vi "Manager.vi"(7 "Action":T1, 8 "Error In":errorcluster, 11 "Set Value":variant) -> (0 "Error Out":errorcluster)   [LabVIEW 2017, in "Logger.lvlib" / "File.lvlib"]
uses:
  File.lvlib
  Action.ctl
  Public/Controls/Statement.ctl
  Public/Controls/Tag.ctl
  Create ISO 8601 File Name.vi
  Write Header.vi
  Create Calendar Folder Tree.vi
  Get Oldest File.vi
  <vilib>/Utility/libraryn.llb/Check if File or Folder Exists.vi
  Create Bulk CSV String.vi
  Logger.lvlib
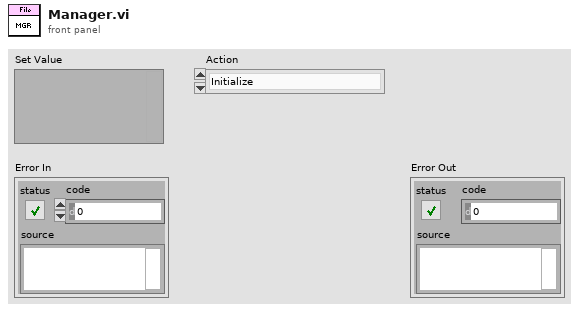
[diagram p1: front panel]
types:
  T1 = typedef "Logger.lvlib/File.lvlib/Action.ctl" = enum16{"Initialize", "Set Maximum File Size", "Set Maximum File Count", "Set Root Folder", "Set Enable Calendar Folder Tree", "Set File Extension", "Start", "Write", "Stop", "Shutdown"}
  T2 = typedef "Logger.lvlib/Statement.ctl" = cluster{"Time Stamp":timestamp, "Tag":T3, "Source":string, "Message":string}
  T3 = typedef "Logger.lvlib/Tag.ctl" = enum16{"Fatal", "Error", "Warn", "Info", "Debug", "Trace"}
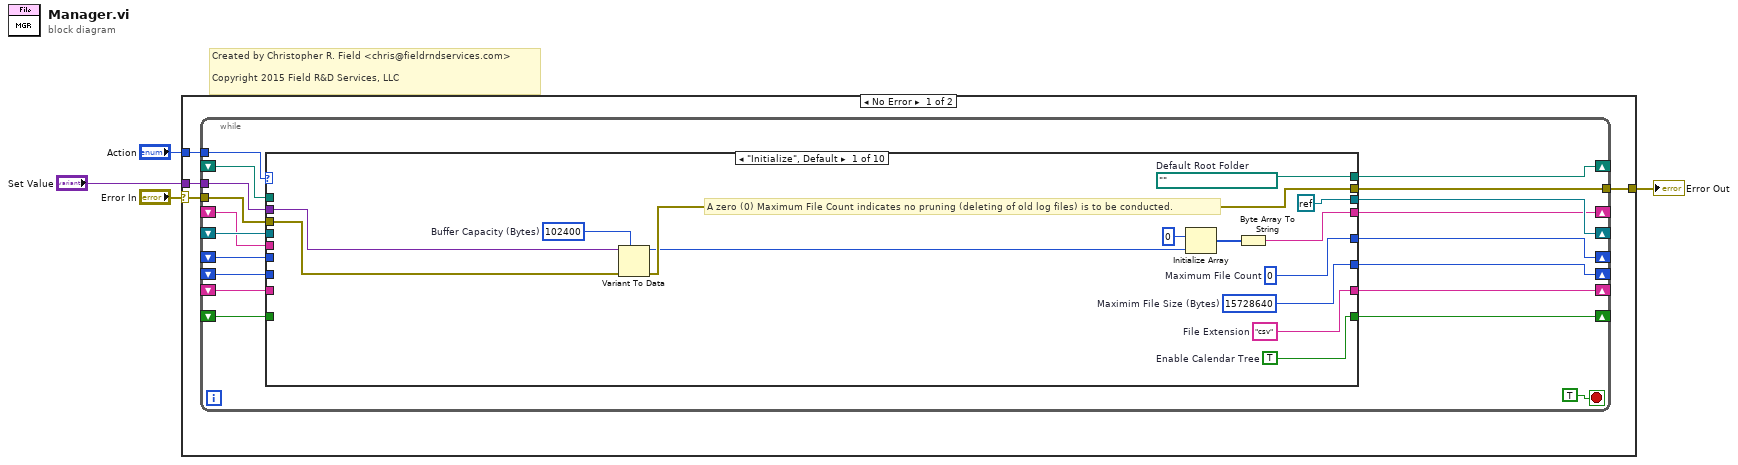
[diagram p0: block diagram]
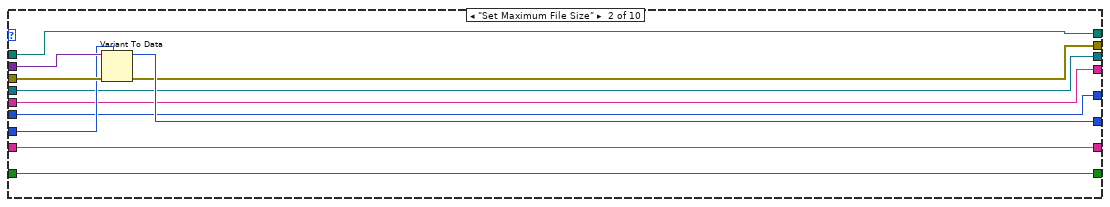
[diagram p2: hidden frame]
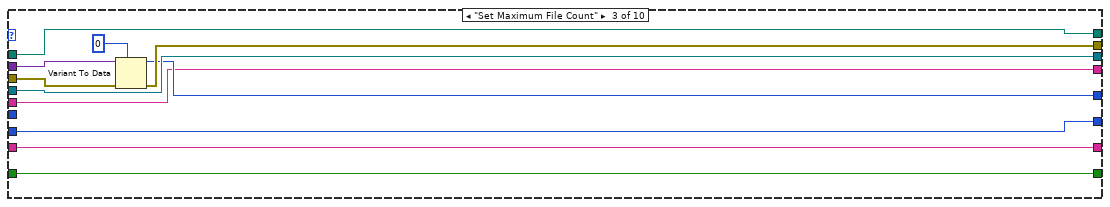
[diagram p3: hidden frame]
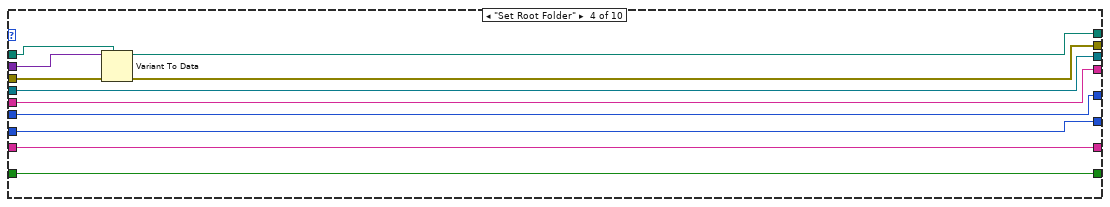
[diagram p4: hidden frame]
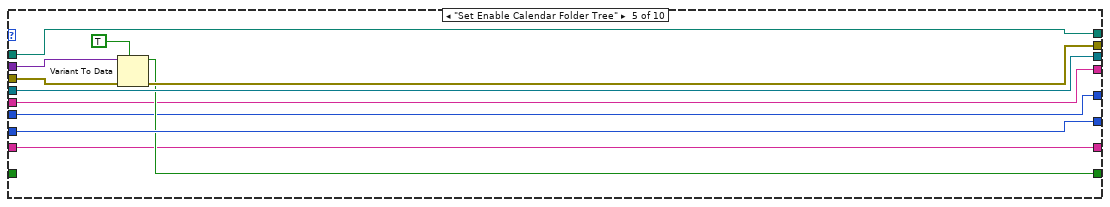
[diagram p5: hidden frame]
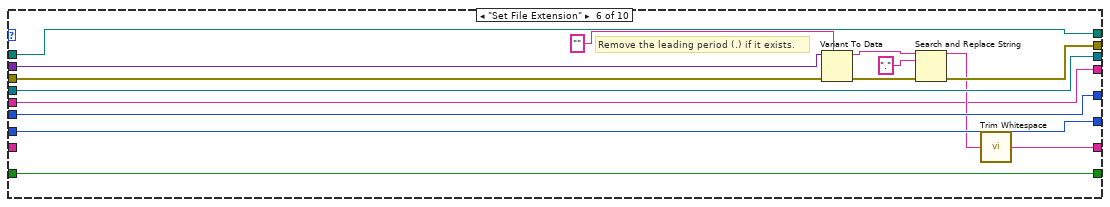
[diagram p6: hidden frame]
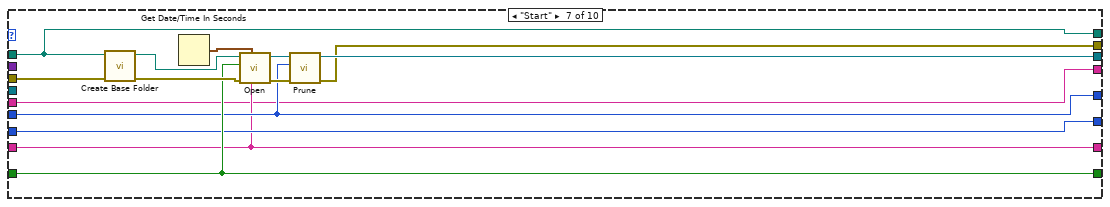
[diagram p7: hidden frame]
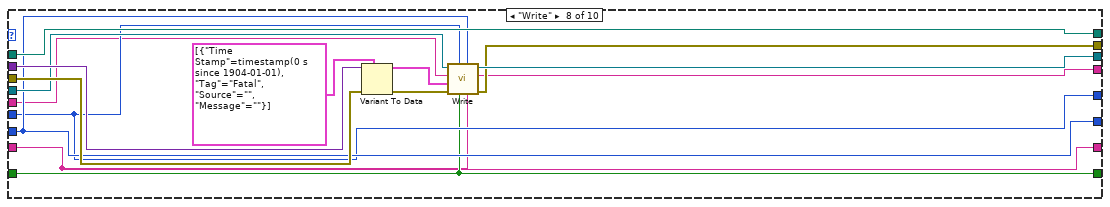
[diagram p8: hidden frame]
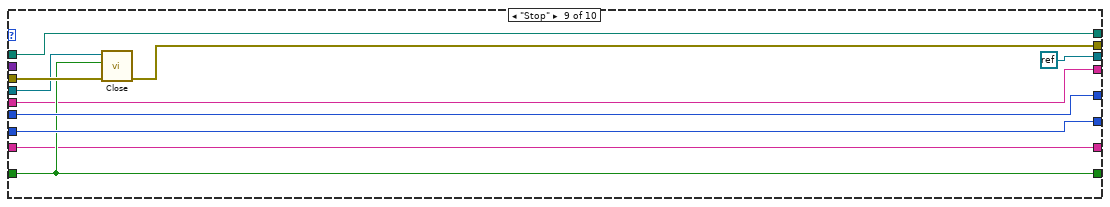
[diagram p9: hidden frame]
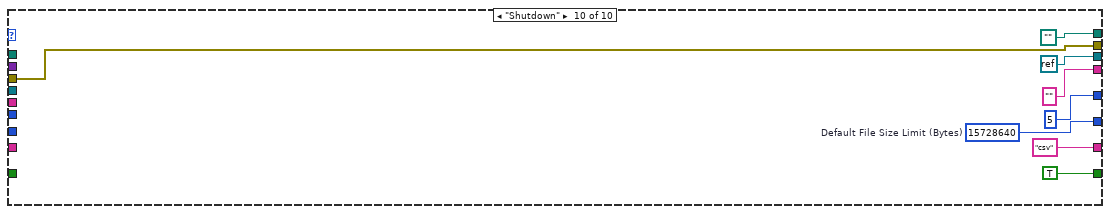
[diagram p10: hidden frame]
diagram:
  # "Created by Christopher R. Field <chris@fieldrndservices.com>\n\nCopyright 2015 Field R&D Services, LLC"
  n1 = case shown="No Error" "Error In" {
    selector: "Error In" -> [w7 w148]
    tunnel: "Action" -> [w8 _]
    tunnel: "Set Value" -> [w6 _]
    tunnel: [w5 w148] -> w1
    frame No Error {
      n2 = while {
        tunnel: w8 -> [w26]
        shift-right: [w25] -> _
        shift-left: _ -> [w20]
        shift-right: [w24] -> _
        shift-left: _ -> [w17]
        shift-right: [w23] -> _
        shift-left: _ -> [w18]
        tunnel: w7 -> [w22]
        tunnel: w6 -> [w21]
        tunnel: [w19] -> w5
        shift-right: [w16] -> _
        shift-left: _ -> [w15]
        shift-right: [w14] -> _
        shift-left: _ -> [w13]
        shift-right: [w12] -> _
        shift-left: _ -> [w11]
        shift-right: [w10] -> _
        shift-left: _ -> [w9]
        stop <- TRUE stop-if-true
        n3 = case shown="\"Initialize\", Default" w26 {
          tunnel: [w41 w49 w57 w74 w85 w100 w104 w121 w135 w144] -> w25
          tunnel: [refnum<k0> refnum w46 w59 w68 w81 w97 w107 w123 refnum<k0> refnum refnum<k0> refnum] -> w24
          tunnel: [w39 w47 w60 w70 w80 w96 w111 w126 w136 path ""] -> w23
          tunnel: w22 -> [w38 w52 w63 w72 w83 w98 w112 w128 w139 w146]
          tunnel: w21 -> [w33 w51 w62 w73 w84 w99 _ w129 _ _]
          tunnel: w20 -> [_ w50 w57 w74 w85 w100 w104 w121 w135 _]
          tunnel: [w34 w48 w61 w69 w82 w91 w105 w122 w134 w146] -> w19
          tunnel: w18 -> [_ w47 w60 w71 w80 w96 w111 w126 w136 _]
          tunnel: w17 -> [_ w46 w59 w68 w81 w97 _ w124 w138 _]
          tunnel: [w37 w45 w58 w67 w78 w93 w108 w116 w132 TRUE] -> w16
          tunnel: w15 -> [_ w45 w58 w67 _ w93 w108 w116 w132 _]
          tunnel: [w36 w44 w55 w66 w77 w95 w103 w120 w133 5] -> w14
          tunnel: w13 -> [_ w44 _ w66 w77 w95 w103 w120 w133 _]
          tunnel: [w35 w43 w54 w65 w76 w87 w102 w115 w131 "csv"] -> w12
          tunnel: w11 -> [_ w43 w54 w65 w76 _ w102 w115 w131 _]
          tunnel: [w28 w42 w53 w64 w75 w86 w101 w119 w130 "" ("Bulk CSV Buffer Out")] -> w10
          tunnel: w9 -> [_ w42 w53 w64 w75 w86 w101 w118 w130 _]
          frame "Initialize", Default {
            w32 = 102400  # Buffer Capacity (Bytes)
            w35 = "csv"  # File Extension
            w36 = 0  # Maximum File Count
            w37 = TRUE  # Enable Calendar Tree
            w39 = path ""  # Default Root Folder
            w41 = i64 15728640  # Maximim File Size (Bytes)
            # "A zero (0) Maximum File Count indicates no pruning (deleting of old log files) is to be conducted."
            n4 = Variant To Data(error in=w38, type=w32, Variant=w33) -> (data=w31:i32, error out=w34:errorcluster)
            n5 = Initialize Array(u8 0, w31) -> (w29:u8[])
            n6 = Byte Array To String(unsigned byte array=w29) -> (string=w28:string)
          }
          frame "Set Maximum File Size" {
            n7 = Variant To Data(error in=w52, type=w50, Variant=w51) -> (data=w49:i64, error out=w48:errorcluster)
          }
          frame "Set Maximum File Count" {
            n8 = Variant To Data(error in=w63, type=0, Variant=w62) -> (data=w55:i32, error out=w61:errorcluster)
          }
          frame "Set Root Folder" {
            n9 = Variant To Data(error in=w72, type=w71, Variant=w73) -> (data=w70:path, error out=w69:errorcluster)
          }
          frame "Set Enable Calendar Folder Tree" {
            n10 = Variant To Data(error in=w83, type=TRUE, Variant=w84) -> (data=w78:bool, error out=w82:errorcluster)
          }
          frame "Set File Extension" {
            # "Remove the leading period (.) if it exists."
            n11 = Variant To Data(error in=w98, type="", Variant=w99) -> (data=w90:string, error out=w92:errorcluster)
            n12 = Search and Replace String(input string=w90, search string=".", error in=w92) -> (result string=w88:string, error out=w91:errorcluster)  [unwired: 5 in, 2 out]
            n13 = call <vilib>:"Trim Whitespace.vi"("string"=w88) -> ("trimmed string"=w87:string)  [unwired: 1 in]
          }
          frame "Start" {
            n14 = call "Create Base Folder.vi"("Error In"=w112, "Root Folder"=w111) -> ("Error Out"=w113:errorcluster, "Base Folder"=w114:path)  [unwired: 8 in]
            n15 = Get Date/Time In Seconds() -> (seconds since 1Jan1904=w109:timestamp)
            n16 = call "Open.vi"("File Extension"=w102, "Start Time Stamp"=w109, "Error In"=w113, "Enable Calendar Tree"=w108, "Base Folder"=w114) -> ("Error Out"=w106:errorcluster, "Log Out"=w110:refnum<file>)  [unwired: 5 in]
            n17 = call "Prune.vi"("Error In"=w106, "Maximum File Count"=w103, "File In"=w110) -> ("Error Out"=w105:errorcluster, "File Out"=w107:refnum<file>)  [unwired: 7 in]
          }
          frame "Write" {
            n18 = Variant To Data(error in=w128, type=T2[] [{"Time Stamp"=timestamp(0 s since 1904-01-01), "Tag"=enum."Fatal", "Source"="", "Message"=""}], Variant=w129) -> (data=w117:T2[], error out=w125:errorcluster)
            n19 = call "Write.vi"("File Extension"=w115, "Maximum File Size (Bytes)"=w121, "Enable Calendar Tree"=w116, "Maximum File Count"=w120, "Error In"=w125, "Messages"=w117, "Bulk CSV Buffer In"=w118, "Log In"=w124) -> ("Error Out"=w122:errorcluster, "Bulk CSV Buffer Out"=w119:string, "Log Out"=w123:refnum<file>)  [unwired: 1 in]
          }
          frame "Stop" {
            n20 = call "Close.vi"("Error In"=w139, "Enable Calendar Tree"=w132, "Log In"=w138) -> ("Error Out"=w134:errorcluster)  [unwired: 7 in, 1 out]
          }
          frame "Shutdown" {
            w144 = i64 15728640  # Default File Size Limit (Bytes)
          }
        }
      }
    }
    frame Error {
    }
  }
  "Error Out" <- w1
